vi "Match 1D String Array.vi"(2 "start index (0)":i32, 3 "Ignore Case? (false)":bool, 4 "Pattern":string, 5 "Strings":string[](array[string])) -> (0 "index of element":i32, 1 "Match":string)   [LabVIEW 2020]
doc: "Searches in <B>Strings</B> for one that matches <B>Pattern</B>.\n\n<B>Pattern</B> - The pattern to search for.\n<B>Strings</B> - The strings to search in.\n<B>start index</B> - The index to start search at.\n<B>Case Sensitive</B> - Honor the case of letters in the pattern.\n<B>index of element</B> - The index of the first matching element.\n<B>Match</B> - The matching element."
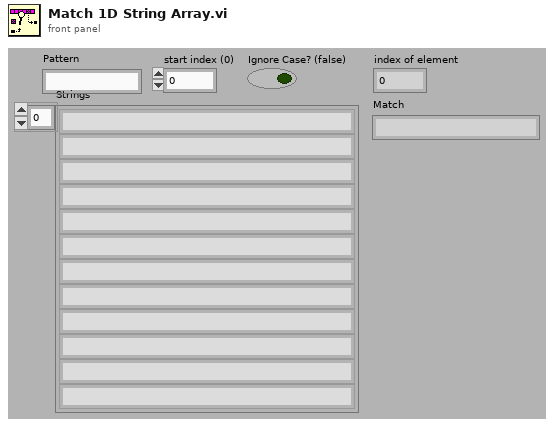
[diagram p1: front panel]
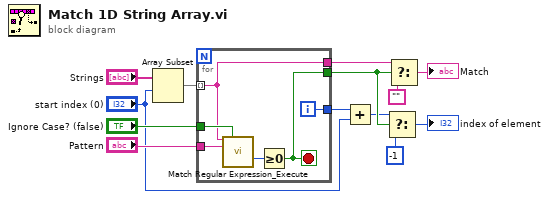
[diagram p0: block diagram]
diagram:
  n1 = Array Subset(array="Strings", index="start index (0)") -> (w12:string[])  [unwired: 1 in]
  n2 = for "Non-Weakly For Loop with Break" {
    tunnel: w12 -> [w15] mode=indexing
    tunnel: "Ignore Case? (false)" -> [w18]
    tunnel: "Pattern" -> [w19]
    tunnel: [w15] -> w5
    tunnel: [w16] -> w6
    tunnel: [w14] -> w3
    i -> [w14]
    stop <- w16 stop-if-true
    n3 = call <vilib>:"Match Regular Expression_Execute.vi"("input string"=w15, "ignore case? (F)"=w18, "regular expression"=w19) -> ("whole match offset"=w17:i32)  [unwired: 7 in, 5 out]
    n4 = Greater Or Equal To 0?(x=w17) -> (x >= 0?=w16:bool)
  }
  n5 = Add(x=w3, y="start index (0)") -> (x+y=w2:i32)
  n6 = Select(t=w2, s=w6, f=-1) -> (s? t:f=→"index of element":i32)
  n7 = Select(t=w5, s=w6, f="") -> (s? t:f=→"Match":string)
